vi "Unicode Multilingual Interface Example.vi"() -> ()   [LabVIEW 2020]
doc: "This example demonstrates reading and displaying unicode text from a file."
uses:
  Types/UTF-8 String/UTF-8 String.lvclass
  Unicode/Controls/String Encoding.ctl
  Types/UTF-8 String/UTF-8 String.lvclass/UTF-8 String.ctl
  Types/UTF-8 Path/UTF-8 Path.lvclass/UTF-8 Path.ctl
  <vilib>/picture/picture.llb/imagedata.ctl
  Dialog & User Interface/Message Box/Message Box Icon Type.ctl
  Dialog & User Interface/Polymorphic VIs/Write Control Text/Write String Value (UTF-8 String).vi
  Dialog & User Interface/Polymorphic VIs/Write Control Text/Write Boolean Text (UTF-8 String).vi
  5a90f179-3b85-4e0c-bde1-5cde268381a4.vi
  26196076-6ab3-4cb0-b291-9633e692300f.vi
  3ad856c3-526a-4e33-8fbe-83f238f9ba6d.vi
  Private/Conversion/Text to UTF-8.vi
  Private/Conversion/Polymorphic VIs/Text to UTF-8 (LabVIEW String).vi
  Dialog & User Interface/Polymorphic VIs/Write Control Text/Write String Value (UTF-8 String).vi/5206cb6b-04fb-41f5-a37e-29c14f142303.vi
  Dialog & User Interface/Polymorphic VIs/Write Control Text/Write Boolean Text (UTF-8 String).vi/5206cb6b-04fb-41f5-a37e-29c14f142303.vi
  Dialog & User Interface/Write Control Caption.vi/13c16a8b-00d3-486b-99f0-c83eae9facb1.vi
  Private/Conversion/String as Encoded String.vi
  Private/Conversion/Polymorphic VIs/String as Encoded String (UTF-8 String).vi
  Types/UTF-8 String/Write Encoded UTF-8 String.vi
  5a90f179-3b85-4e0c-bde1-5cde268381a4.vi/9afeabe8-8abe-4536-bea1-05e5a3549c28.vi
  Private/Conversion/Text as Encoded String.vi
  Private/Conversion/Polymorphic VIs/Text as Encoded String (UTF-8 Path).vi
  Private/Library/gu_open_file_dialog.vi
  Private/Library/gu_select_folder_dialog.vi
  26196076-6ab3-4cb0-b291-9633e692300f.vi/c24c063b-f849-48a1-b323-238a063d7118.vi
  26196076-6ab3-4cb0-b291-9633e692300f.vi/a2fd6c11-d594-45c9-8624-1f0a1df69df3.vi
  26196076-6ab3-4cb0-b291-9633e692300f.vi/1fd3173e-d32e-42cb-8f0d-819132eb8e27.vi
  26196076-6ab3-4cb0-b291-9633e692300f.vi/bb7c39fc-ad8e-447d-bc50-468674bfb562.vi
  Private/Conversion/Path as UTF-8 Path.vi
  Private/Conversion/Polymorphic VIs/Path as UTF-8 Path (UTF-8 Path).vi
  Private/Conversion/Polymorphic VIs/Text as Encoded String (UTF-8 String).vi
  Private/Conversion/Text as Encoded Path.vi
  Private/Conversion/Polymorphic VIs/Text as Encoded Path (UTF-8 String).vi
  Types/UTF-8 Path/Write Encoded UTF-8 Path.vi
  Types/UTF-8 Path/Read Encoded UTF-8 Path.vi
  Private/Memory/Copy String.vi
  Private/Library/Result To Error.vi
  Private/Conversion/Path as Encoded Path.vi
  Private/Conversion/Polymorphic VIs/Path as Encoded Path (UTF-8 Path).vi
  Private/Library/gu_string_subset.vi
  Private/Library/gu_to_lower_case.vi
  Private/Library/gu_search_split_string.vi
  Private/Conversion/Polymorphic VIs/String as Encoded String (LabVIEW String).vi
  Private/Memory/Copy String.vi/4d47babd-4a2d-4eb7-b91b-7e707d692665.vi
  Private/Library/gu_free.vi
  <vilib>/Utility/config.llb/Read Key (String).vi
  Unicode/Detect String Encoding.vi
  Private/Conversion/Encoded UTF-16LE String to Encoded UTF-8 String.vi
  Private/Conversion/Encoded UTF-8 String to Encoded UTF-16LE String.vi
  Private/User Interface/Write String.vi
  Private/User Interface/Write Boolean Text.vi
  Private/User Interface/Write Caption.vi
  <vilib>/Utility/error.llb/Error Cluster From Error Code.vi
  Private/Library/gu_message_box.vi
  Types/UTF-8 Path/UTF-8 Path.lvclass
  <vilib>/Utility/config.llb/NI_LVConfig.lvlib
  G-Unicode.lvlib
panel:
  in  "Language":u16(ring) items=["english", "arabic", "chinese", "japanese", "korean", "polish", "russian", "thai"]
  in  "button":bool caption="¹0¤0Ã0Á0"
  out "message":string="Hello. Here is the interface in English."
  out "height":i16 caption="Height"
  out "width":i16 caption="Width"
  out "image":picture caption="Image"
  # "Instructions:\n1. Run the VI.\n2. Select a language from the text ring. The UI will update to display in that language.\n3. Click the Open File button and select an image file (note the file dialog title is also translated).\n4. The image will be loaded. If a non-image file was selected, a translated error message dialog is displayed."
  # "G"
  # "-Unicode"
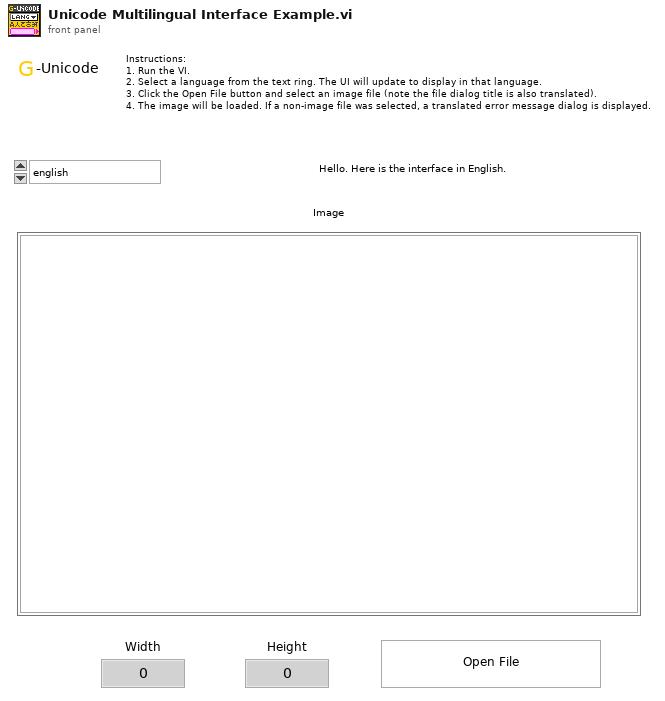
[diagram p1: front panel]
types:
  T1 = map{string, map{string, refnum<class "UTF-8 String.lvclass">}}
  T2 = typedef "NI_LVConfig.lvlib/Config Data RefNum.ctl" = refnum<k1>
  T3 = map{string, refnum<class "UTF-8 String.lvclass">}
  T4 = typedef "G-Unicode.lvlib/String Encoding.ctl" = enum16{"ANSI", "UTF-8", "UTF-16LE", "UTF-16BE", "Unknown"}
  T5 = typedef "G-Unicode.lvlib/Message Box Icon Type.ctl" = enum16{"Info", "Warning", "Error", "Question"}
  T6 = typedef "imagedata.ctl" = cluster{"image type":i32, "image depth":i32, "image":u8[], "mask":u8[], "colors":u32[], "Rectangle":cluster{"left":i16, "top":i16, "right":i16, "bottom":i16}}
  T7 = typedef "G-Unicode.lvlib/Encoded UTF-8 String.ctl" = string
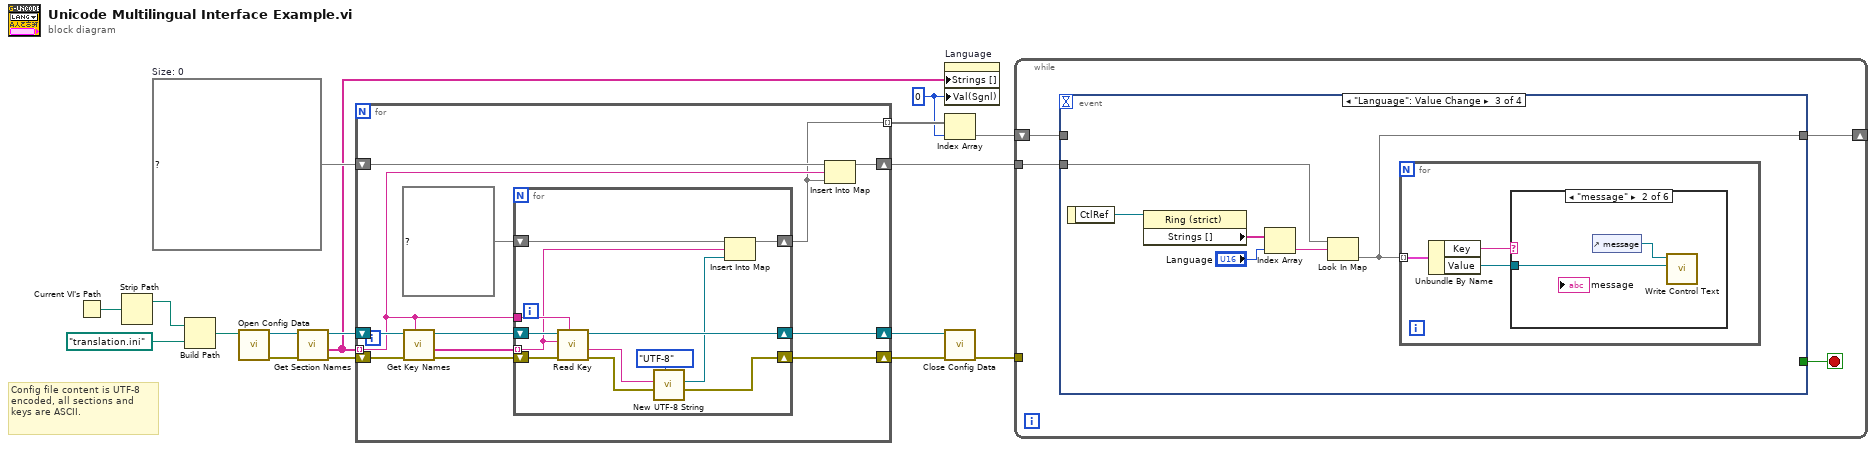
[diagram p0: block diagram]
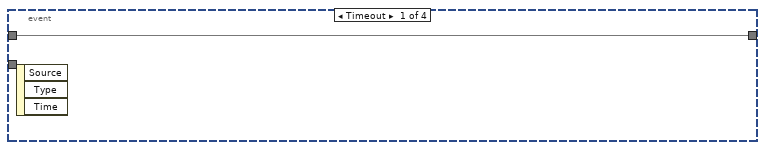
[diagram p2: hidden frame]
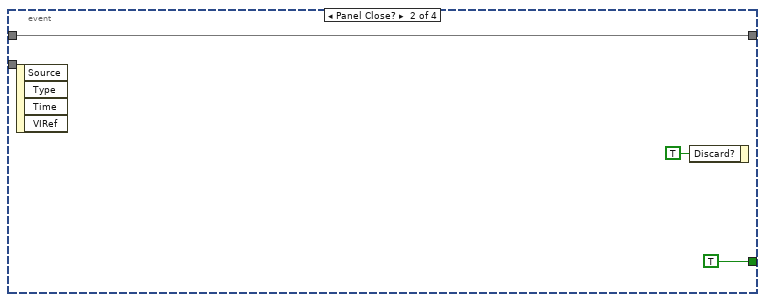
[diagram p3: hidden frame]
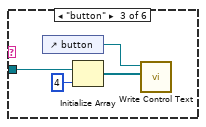
[diagram p5: hidden frame]
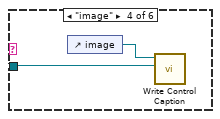
[diagram p6: hidden frame]
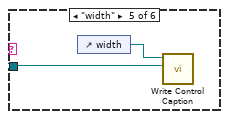
[diagram p7: hidden frame]
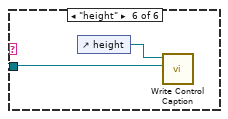
[diagram p8: hidden frame]
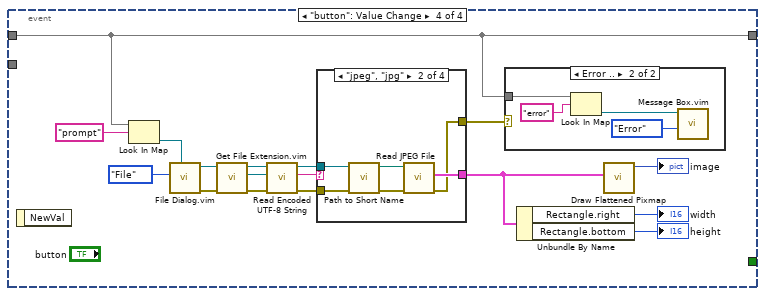
[diagram p9: hidden frame]
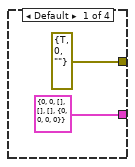
[diagram p11: hidden frame]
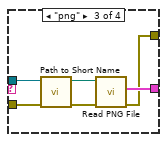
[diagram p12: hidden frame]
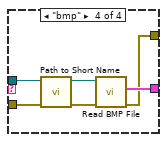
[diagram p13: hidden frame]
diagram:
  w1 = u16 0 ("Value (Signaling)")
  w11 = T1 {}  # Size: 0
  # "Config file content is UTF-8 encoded, all sections and keys are ASCII."
  n1 = Current VI's Path() -> (path=w10:path)
  n2 = Strip Path(path=w10) -> (stripped path=w8:path)  [unwired: 1 out]
  n3 = Build Path(base path=w8, name or relative path=path "translation.ini") -> (appended path=w7:path)
  n4 = call <vilib>:"Open Config Data.vi"("configuration file path"=w7) -> ("error out"=w13:errorcluster, "refnum"=w17:T2)  [unwired: 8 in, 1 out]
  n5 = call <vilib>:"Get Section Names.vi"("error in (no error)"=w13, "refnum"=w17) -> ("error out"=w14:errorcluster, "section names"=w2:string[], "refnum out"=w16:T2)  [unwired: 7 in]
  n6 = for {
    tunnel: w2 -> [w20] mode=indexing
    shift-right: [w26] -> w15
    shift-left: w16 -> [w29]
    shift-right: [w25] -> w12
    shift-left: w14 -> [w24]
    shift-right: [w22] -> w5
    shift-left: w11 -> [w21]
    tunnel: [w18] -> w3 mode=indexing
    n7 = call <vilib>:"Get Key Names.vi"("section"=w20, "error in (no error)"=w24, "refnum"=w29) -> ("error out"=w23:errorcluster, "key names"=w28:string[], "refnum out"=w27:T2)  [unwired: 5 in, 1 out]
    n8 = for {
      tunnel: w28 -> [w32] mode=indexing
      shift-right: [w40] -> w26
      shift-left: w27 -> [w41]
      tunnel: w20 -> [w38]
      shift-right: [w35] -> w25
      shift-left: w23 -> [w34]
      shift-right: [w30] -> w18
      shift-left: T3 {} ("Translation") -> [w33]
      n9 = call-poly <vilib>:"Read Key.vi"("section"=w38, "error in (no error)"=w34, "key"=w32, "refnum"=w41) -> ("error out"=w36:errorcluster, "value"=w37:string, "refnum out"=w40:T2)  [unwired: 4 in, 1 out]
      n10 = call "New UTF-8 String.vi"("Input Encoding (ANSI)"=String_Encoding."UTF-8", "error in"=w36, "String"=w37) -> ("error out"=w35:errorcluster, "UTF-8 String"=w31:refnum<class "UTF-8 String.lvclass">)  [unwired: 7 in]
      n11 = Insert Into Map(map in=w33, key=w32, value=w31) -> (map out=w30:T3)  [unwired: 2 out]
    }
    n12 = Insert Into Map(map in=w21, key=w20, value=w18) -> (map out=w22:T1)  [unwired: 2 out]
  }
  n13 = property on="Language" class="Ring (strict)"("Strings []"=w2, "Val(Sgnl)"=w1) -> ()  [unwired: 2 in, 2 out]
  n14 = Index Array(array=w3, index=w1) -> (element=w4:T3)
  n15 = call <vilib>:"Close Config Data.vi"("error in (no error)"=w12, "refnum"=w15) -> ("error out"=w6:errorcluster)  [unwired: 8 in, 1 out]
  n16 = while {
    tunnel: w5 -> [w45]
    tunnel: w6 -> [_]
    shift-right: [w44] -> _
    shift-left: w4 -> [w43]
    stop <- w42 stop-if-true
    n17 = event shown="[2] \"Language\": Value Change" {
      selector: _ -> [_ _ _ _]
      dyn-events: _ -> [_ _ _ _]
      timeout: _ -> [_ _ _ _]
      tunnel: w45 -> [_ _ w55 _]
      tunnel: [w46 w49 w51 w73] -> w44
      tunnel: w43 -> [w46 w49 _ w73]
      tunnel: [_ TRUE _ _] -> w42
      event Timeout {
        n18 = event-data() -> ()  [unwired: 1 in, 3 out]
      }
      event Panel Close? {
        n19 = event-data() -> ()  [unwired: 1 in, 4 out]
        n20 = event-data("Discard?"=TRUE) -> ()  [unwired: 1 in, 1 out]
      }
      event "Language": Value Change {
        n21 = event-data() -> ("CtlRef"=w54:refnum<vi>)  [unwired: 1 in]
        n22 = property class="Ring (strict)"(reference=w54) -> ("Strings []"=w53:string[])  [unwired: 1 in, 2 out]
        n23 = Index Array(array=w53, index="Language") -> (element=w52:string)
        n24 = Look In Map(map=w55, key=w52) -> (value=w51:T3)  [unwired: 1 in, 1 out]
        n25 = for {
          tunnel: w51 -> [w58] mode=indexing
          n26 = Unbundle By Name(w58) -> ("Key"=w57:string, "Value"=w56:refnum<class "UTF-8 String.lvclass">)
          n27 = case shown="\"message\"" w57 {
            tunnel: w56 -> [_ w59 w64 w65 w68 w70]
            frame Default {
            }
            frame "message" {
              n28 = control-ref of="message"() -> (w60:refnum<vi>)
              n29 = call-poly "Write Control Text.vi"("Value"=w59, "Control Ref"=w60) -> ()  [unwired: 9 in, 1 out]
            }
            frame "button" {
              n30 = control-ref of="button"() -> (w61:refnum<vi>)
              n31 = Initialize Array(w64, 4 ("dimension size")) -> (w62:refnum<class "UTF-8 String.lvclass">[])
              n32 = call-poly "Write Control Text.vi"("Value"=w62, "Control Ref"=w61) -> ()  [unwired: 9 in, 1 out]
            }
            frame "image" {
              n33 = control-ref of="image"() -> (w66:refnum<vi>)
              n34 = call "Write Control Caption.vi"("Text"=w65, "Control Ref"=w66) -> ()  [unwired: 9 in, 1 out]
            }
            frame "width" {
              n35 = control-ref of="width"() -> (w67:refnum<vi>)
              n36 = call "Write Control Caption.vi"("Text"=w68, "Control Ref"=w67) -> ()  [unwired: 9 in, 1 out]
            }
            frame "height" {
              n37 = control-ref of="height"() -> (w69:refnum<vi>)
              n38 = call "Write Control Caption.vi"("Text"=w70, "Control Ref"=w69) -> ()  [unwired: 9 in, 1 out]
            }
          }
        }
      }
      event "button": Value Change {
        n39 = event-data() -> ()  [unwired: 1 in, 1 out]
        n40 = Look In Map(map=w73, key="prompt") -> (value=w74:refnum<class "UTF-8 String.lvclass">)  [unwired: 1 in, 1 out]
        n41 = call "File Dialog.vim"("Prompt"=w74, "Selection"=enum16{"File", "Multiple Files", "Folder"}."File") -> ("error out"=w72:errorcluster, "Selected Path"=w84:refnum<class "UTF-8 Path.lvclass">)  [unwired: 7 in, 1 out]
        n42 = call "Get File Extension.vim"("error in (no error)"=w72, "file"=w84) -> ("error out"=w71:errorcluster, "lowercase file extension"=w83:refnum<class "UTF-8 String.lvclass">, "dup file"=w81:refnum<class "UTF-8 Path.lvclass">)  [unwired: 5 in, 2 out]
        n43 = call "Read Encoded UTF-8 String.vi"("UTF-8 String"=w83) -> ("Encoded UTF-8 String"=w82:T7)  [unwired: 10 in]
        n44 = case shown="\"jpeg\", \"jpg\"" w82 {
          tunnel: w81 -> [_ w97 w103 w109]
          tunnel: [T6 {"image type"=0, "image depth"=0, "image"=[], "mask"=[], "colors"=[], "Rectangle"={"left"=0, "top"=0, "right"=0, "bottom"=0}} ("image data") w95 w101 w107] -> w79
          tunnel: [errorcluster {"status"=TRUE, "code"=0, "source"=""} ("error out") w94 w100 w106] -> w76
          tunnel: w71 -> [_ w92 w99 w105]
          frame Default {
          }
          frame "jpeg", "jpg" {
            n45 = call "Path to Short Name.vi"("error in"=w92, "Path"=w97) -> ("error out"=w93:errorcluster, "LabVIEW Path"=w96:path)  [unwired: 8 in]
            n46 = call <vilib>:"Read JPEG File.vi"("error in (no error)"=w93, "path to JPEG file"=w96) -> ("error out"=w94:errorcluster, "image data"=w95:T6)  [unwired: 7 in, 1 out]
          }
          frame "png" {
            n47 = call "Path to Short Name.vi"("error in"=w99, "Path"=w103) -> ("error out"=w98:errorcluster, "LabVIEW Path"=w102:path)  [unwired: 8 in]
            n48 = call <vilib>:"Read PNG File.vi"("error in (no error)"=w98, "path to PNG file"=w102) -> ("error out"=w100:errorcluster, "image data"=w101:T6)  [unwired: 7 in, 1 out]
          }
          frame "bmp" {
            n49 = call "Path to Short Name.vi"("error in"=w105, "Path"=w109) -> ("error out"=w104:errorcluster, "LabVIEW Path"=w108:path)  [unwired: 8 in]
            n50 = call <vilib>:"Read BMP File.vi"("error in (no error)"=w104, "path to BMP file"=w108) -> ("error out"=w106:errorcluster, "image data"=w107:T6)  [unwired: 7 in, 1 out]
          }
        }
        n51 = case shown="Error .." w76 {
          tunnel: w73 -> [_ w87]
          frame No Error {
          }
          frame Error {
            n52 = Look In Map(map=w87, key="error") -> (value=w86:refnum<class "UTF-8 String.lvclass">)  [unwired: 1 in, 1 out]
            n53 = call "Message Box.vim"("Icon (Info)"=Message_Box_Icon_Type."Error", "Message"=w86) -> ()  [unwired: 8 in, 2 out]
          }
        }
        n54 = Unbundle By Name(w79) -> ("Rectangle.right"=→"width":i16, "Rectangle.bottom"=→"height":i16)
        n55 = call <vilib>:"Draw Flattened Pixmap.vi"("image data"=w79) -> ("new picture"=→"image":picture)  [unwired: 8 in]
      }
    }
  }
